vi "FileIO_Sequence_Replace_ERDNumbers_With_Names.vi"() -> ()   [LabVIEW 2016]
doc: "This VI will take a TestStand Sequence File (must be saved as ini file) and replace ERD # (e.g. 0xF000) with the ERD Variable name from the firmware generated XML file. Numbers are replaced with FileGlobals.ERDs.ERD_Name\n\nMust have an ERD Defintions XML file for your project.\n\nAlso, before running all references to ERD must be in hex numeric format (e.g. 0xF000), must remove any fileglobals or ERD numbers saved as variables throughout the seq.\n\nAfter running you can run the common code to add fileglobals to the sequence."
panel:
  in  "Seq Path In":path
  out "Seq Path Out":path
  in  "ERD XML File":path
  in  "Error In":errorcluster
  out "error out":errorcluster
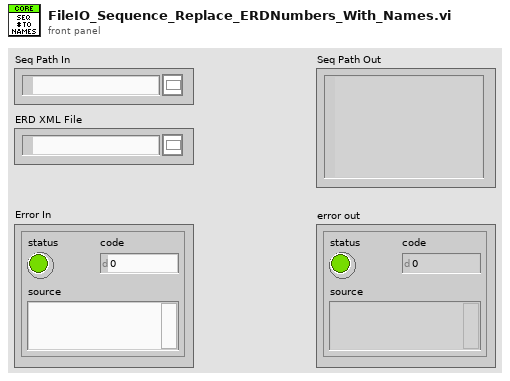
[diagram p1: front panel]
types:
  T1 = enum16{"open", "replace", "create", "open or create", "replace or create", "replace or create with confirmation"}
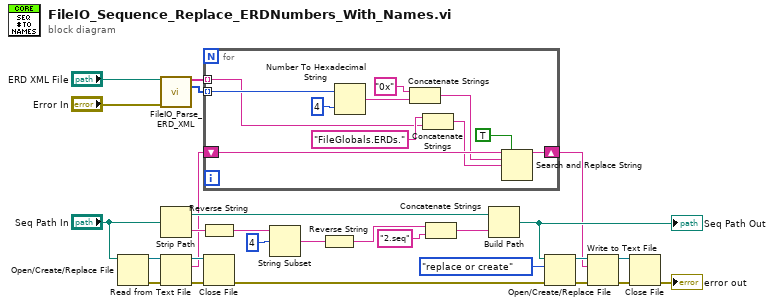
[diagram p0: block diagram]
diagram:
  n1 = Open/Create/Replace File(file path (use dialog)="Seq Path In") -> (refnum out=w27:refnum<file>, error out=w26:errorcluster)  [unwired: 5 in, 1 out]
  n2 = call "FileIO_Parse_ERD_XML.vi"("ERD XML File"="ERD XML File", "Error In"="Error In") -> ("ERD Names"=w4:string[], "ERD Numbers"=w3:u16[])  [unwired: 10 in, 2 out]
  n3 = Strip Path(path="Seq Path In") -> (stripped path=w14:path, name=w22:string)
  n4 = Read from Text File(file (use dialog)=w27, error in=w26) -> (refnum out=w25:refnum<file>, text=w7:string, error out=w24:errorcluster)  [unwired: 2 in, 1 out]
  n5 = for {
    shift-right: [w36] -> w6
    shift-left: w7 -> [w37]
    tunnel: w3 -> [w34] mode=indexing
    tunnel: w4 -> [w29] mode=indexing
    n6 = Number To Hexadecimal String(1:i16 4 ("width (-)"), 2:w34) -> (0:w33:string)
    n7 = Concatenate Strings("0x", w33) -> (w31:string)
    n8 = Concatenate Strings("FileGlobals.ERDs." ("string"), w29) -> (w28:string)
    n9 = Search and Replace String(replace all?=TRUE ("replace all? (F)"), input string=w37, search string=w31, replace string=w28) -> (result string=w36:string)  [unwired: 4 in, 3 out]
  }
  n10 = Reverse String(1:w22) -> (0:w21:string)
  n11 = Close File(refnum=w25, error in=w24) -> (error out=w23:errorcluster)  [unwired: 1 out]
  n12 = String Subset(string=w21, offset (0)=4) -> (substring=w19:string)  [unwired: 1 in]
  n13 = Reverse String(1:w19) -> (0:w18:string)
  n14 = Concatenate Strings(w18, "2.seq" ("string")) -> (w16:string)
  n15 = Build Path(base path=w14, name or relative path=w16) -> (appended path=w13:path)
  "Seq Path Out" <- w13
  n16 = Open/Create/Replace File(file path (use dialog)=w13, error in=w23, operation (0:open)=T1."replace or create") -> (refnum out=w11:refnum<file>, error out=w12:errorcluster)  [unwired: 3 in, 1 out]
  n17 = Write to Text File(file (use dialog)=w11, text=w6, error in=w12) -> (refnum out=w9:refnum<file>, error out=w10:errorcluster)  [unwired: 1 in, 1 out]
  n18 = Close File(refnum=w9, error in=w10) -> (error out=→"error out":errorcluster)  [unwired: 1 out]
